vi "Calculate Particle Scores2.vi"(10 "Sorted Data":dbl[][](array[numeric]), 11 "Good":bool) -> (3 "Scores":T2[](array[typedef]))   [LabVIEW 2019]
doc: "Calculate scores based on the particle measurements. Calculated scores are for aspect ratio, area to convex hull area, and moment of inertia. These scores range between 0 and 100 and can be used to categorize particles as targets and non-targets."
uses:
  Target Fields.ctl
  <vilib>/Analysis/baseanly.llb/Mean (DBL).vi
  <vilib>/Analysis/NI_AALBase.lvlib
panel:
  out "Array":T1(array[cluster])
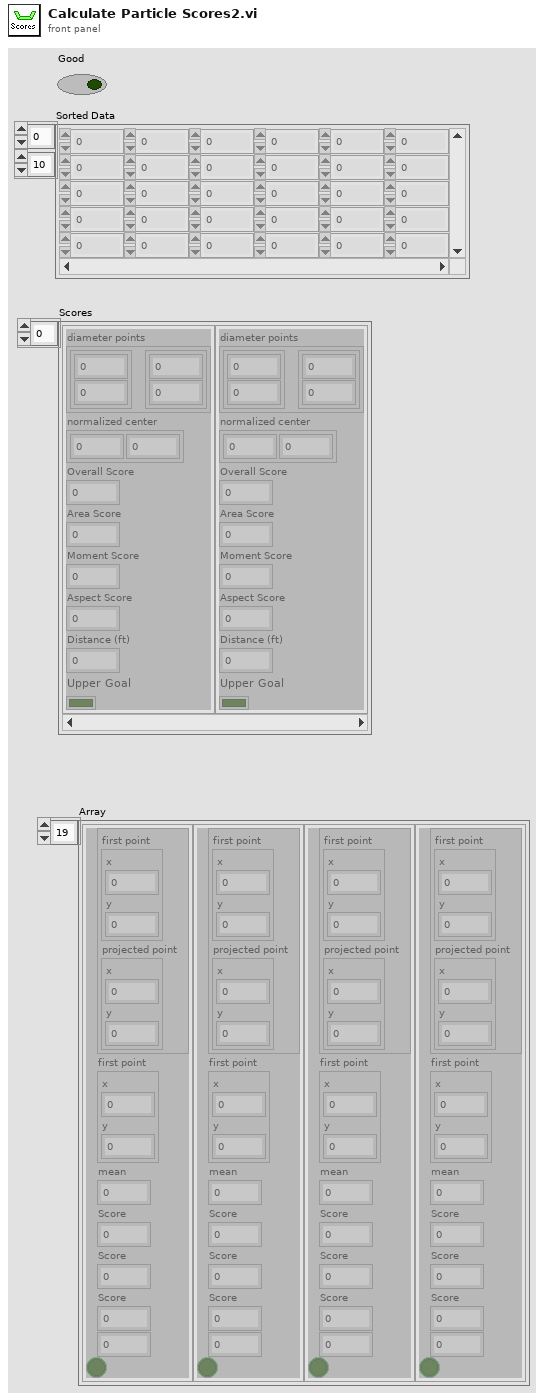
[diagram p1: front panel]
types:
  T1 = cluster{cluster{"first point":cluster{"x":dbl, "y":dbl}, "projected point":cluster{"x":dbl, "y":dbl}}, "first point":cluster{"x":dbl, "y":dbl}, "mean":dbl, "Score":dbl, "Score":dbl, "Score":dbl, dbl, bool}[]
  T2 = typedef "Target Fields.ctl" = cluster{"diameter points":cluster{"first point":cluster{"x":dbl, "y":dbl}, "projected point":cluster{"x":dbl, "y":dbl}}, "normalized center":cluster{"x":dbl, "y":dbl}, "Overall Score":dbl, "Area Score":dbl, "Moment Score":dbl, "Aspect Score":dbl, "Distance (ft)":dbl, "Upper Goal":bool}
  T3 = cluster{cluster{"Numeric":dbl, "Numeric":dbl}, cluster{"Numeric":dbl, "Numeric":dbl}}
  T4 = cluster{"first point":cluster{"x":dbl, "y":dbl}, "projected point":cluster{"x":dbl, "y":dbl}}
  T5 = cluster{cluster{"first point":cluster{"x":dbl, "y":dbl}, "projected point":cluster{"x":dbl, "y":dbl}}, "first point":cluster{"x":dbl, "y":dbl}, "mean":dbl, "Score":dbl, "Score":dbl, "Score":dbl, dbl, bool}
  T6 = cluster{cluster{cluster{"Numeric":dbl, "Numeric":dbl}, cluster{"Numeric":dbl, "Numeric":dbl}}, "first point":cluster{"x":dbl, "y":dbl}, "mean":dbl, "Score":dbl, "Score":dbl, "Score":dbl, dbl, bool}
  T7 = cluster{cluster{"first point":cluster{"Numeric":dbl, "Numeric":dbl}, "projected point":cluster{"Numeric":dbl, "Numeric":dbl}}, "first point":cluster{"x":dbl, "y":dbl}, "mean":dbl, "Score":dbl, "Score":dbl, "Score":dbl, dbl, bool}
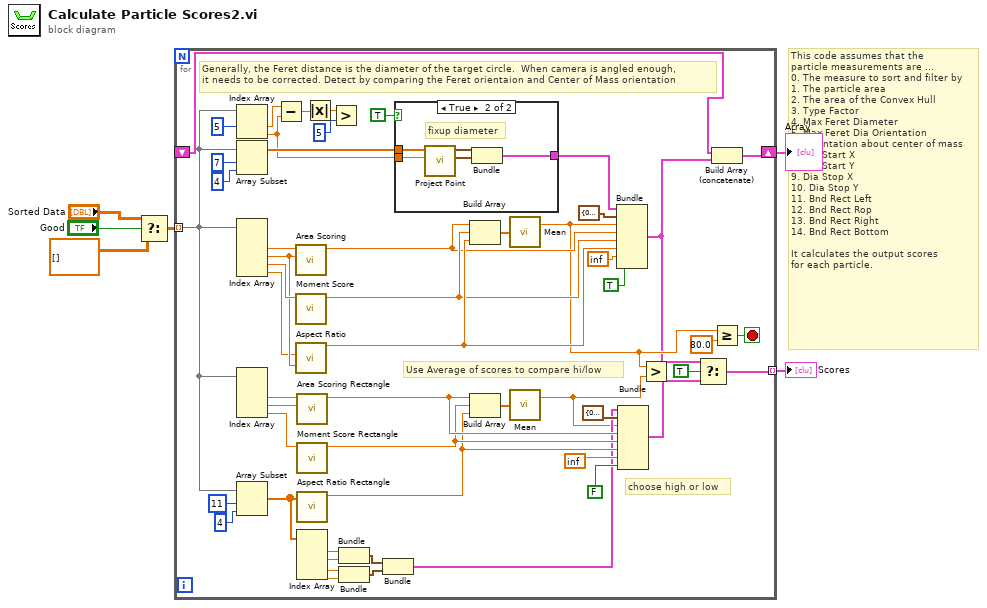
[diagram p0: block diagram]
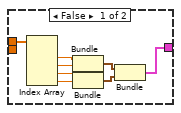
[diagram p2: hidden frame]
diagram:
  # "This code assumes that the\nparticle measurements are ...\n0. The measure to sort and filter by\n1. The particle area\n2. The area of the Convex Hull\n3. Type Factor\n4. Max Feret Diameter\n5. Max Feret Dia Orientation\n6. Orientation about center of mass\n7. Dia Start X\n8. Dia Start Y\n9. Dia Stop X\n10. Dia Stop Y\n11. Bnd Rect Left\n12. Bnd Rect Rop\n13. Bnd Rect Right\n14. Bnd Rect Bottom\n\nIt calculates the output scores\nfor each particle."
  n1 = Select(t="Sorted Data", s="Good", f=dbl[][] []) -> (s? t:f=w2:dbl[][])
  n2 = for {
    tunnel: w2 -> [w19] mode=indexing
    tunnel: [w33] -> w6 mode=indexing
    shift-right: [w10] -> w1
    shift-left: _ -> [w8]
    stop <- w15 stop-if-true
    # "Use Average of scores to compare hi/low"
    # "choose high or low"
    # "Generally, the Feret distance is the diameter of the target circle.  When camera is angled enough,\nit needs to be corrected. Detect by comparing the Feret orientaion and Center of Mass orientation"
    n3 = Index Array(array=w19, index #1=5 ("index")) -> (element #1=w52:dbl, element #2=w47:dbl)  [unwired: 1 in]
    n4 = Array Subset(array=w19, index=7, length=4) -> (w48:dbl[])
    n5 = Index Array(array=w19) -> (element #2=w59:dbl, element #3=w57:dbl, element #4=w58:dbl, element #5=w56:dbl)  [unwired: 5 in, 1 out]
    n6 = Index Array(array=w19) -> (element #2=w39:dbl, element #3=w38:dbl, element #4=w37:dbl)  [unwired: 4 in, 1 out]
    n7 = Array Subset(array=w19, index=11, length=4) -> (w18:dbl[])
    n8 = Subtract(x=w52, y=w47) -> (x-y=w55:dbl)
    n9 = call "Area Scoring.vi"("Convex Hull Area"=w57, "Area"=w59) -> ("Score"=w43:dbl)  [unwired: 9 in]
    n10 = call "Moment Score.vi"("Moment Factor"=w58) -> ("Score"=w44:dbl)  [unwired: 10 in]
    n11 = call "Aspect Ratio.vi"("Diameter"=w56, "Convex Hull Area"=w57) -> ("Score"=w45:dbl)  [unwired: 9 in]
    n12 = call "Area Scoring Rectangle.vi"("Convex Hull Area"=w38, "Area"=w39) -> ("Score"=w31:dbl)  [unwired: 9 in]
    n13 = call "Moment Score Rectangle.vi"("Moment Factor"=w37) -> ("Score"=w30:dbl)  [unwired: 10 in]
    n14 = call "Aspect Ratio Rectangle.vi"("Bounds"=w18) -> ("Score"=w29:dbl)  [unwired: 10 in]
    n15 = Index Array(array=w18) -> (element #1=w26:dbl, element #2=w25:dbl, element #3=w24:dbl, element #4=w23:dbl)  [unwired: 4 in]
    n16 = Absolute Value(x=w55) -> (abs(x)=w53:dbl)
    n17 = Greater?(x=w53, y=5 ("length")) -> ()  [unwired: 1 out]
    n18 = Bundle("Numeric"=w26, "Numeric"=w25) -> (w22:cluster{"Numeric":dbl, "Numeric":dbl})  [unwired: 1 in]
    n19 = Bundle("Numeric"=w24, "Numeric"=w23) -> (w21:cluster{"Numeric":dbl, "Numeric":dbl})  [unwired: 1 in]
    n20 = Bundle(w22, w21) -> (w20:T3)  [unwired: 1 in]
    n21 = case shown="True" TRUE {
      tunnel: w48 -> [w65 w72]
      tunnel: w47 -> [_ w71]
      tunnel: [w60 w68] -> w42
      frame False {
        n22 = Index Array(array=w65) -> (element #1=w63:dbl, element #2=w64:dbl, element #3=w66:dbl, element #4=w67:dbl)  [unwired: 4 in]
        n23 = Bundle("Numeric"=w63, "Numeric"=w64) -> (w62:cluster{"Numeric":dbl, "Numeric":dbl})  [unwired: 1 in]
        n24 = Bundle("Numeric"=w66, "Numeric"=w67) -> (w61:cluster{"Numeric":dbl, "Numeric":dbl})  [unwired: 1 in]
        n25 = Bundle(w62, w61) -> (w60:T3)  [unwired: 1 in]
      }
      frame True {
        # "fixup diameter"
        n26 = call "Project Point.vi"("orientation (deg)"=w71, "coordinates"=w72) -> ("projected point"=w69:cluster{"x":dbl, "y":dbl}, "first point"=w70:cluster{"x":dbl, "y":dbl})  [unwired: 8 in]
        n27 = Bundle("first point"=w70, "projected point"=w69) -> (w68:T4)  [unwired: 1 in]
      }
    }
    n28 = Build Array(w43, w44, w45) -> (w14:dbl[])
    n29 = Build Array(w31, w30, w29) -> (w13:dbl[])
    n30 = call-poly <vilib>:"Mean.vi"("X"=w14) -> ("mean"=w17:dbl)  [unwired: 1 out]
    n31 = call-poly <vilib>:"Mean.vi"("X"=w13) -> ("mean"=w12:dbl)  [unwired: 1 out]
    n32 = Bundle(w42, "first point"=cluster{"x":dbl, "y":dbl} {"x"=0.0, "y"=0.0}, "mean"=w17, "Score"=w43, "Score"=w44, "Score"=w45, inf, TRUE) -> (w9:T5)  [unwired: 1 in]
    n33 = Bundle(w20, "first point"=cluster{"x":dbl, "y":dbl} {"x"=0.0, "y"=0.0}, "mean"=w12, "Score"=w31, "Score"=w30, "Score"=w29, inf, FALSE) -> (w34:T6)  [unwired: 1 in]
    n34 = Greater?(x=w17, y=w12) -> ()  [unwired: 1 out]
    n35 = Select(t=w9, s=TRUE, f=w34) -> (s? t:f=w33:T7)
    n36 = Build Array (concatenate)(w8, w9) -> (w10:T1)
    n37 = Greater Or Equal?(x=w17, y=80.0) -> (x >= y?=w15:bool)
  }
  "Scores" <- w6
  "Array" <- w1
